vi "Julian Day_subVI.vi"() -> (0 "second":dbl, 1 "minute":dbl, 2 "hour":dbl, 3 "Julian Day":dbl format="%#_8g")   [LabVIEW 2019]
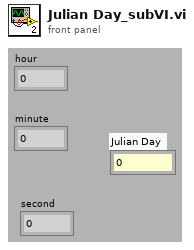
[diagram p1: front panel]
types:
  T1 = cluster{"second":i32, "minute":i32, "hour":i32, "day of month":i32, "month":i32, "year":i32, "day of week":i32, "day of year":i32, "is DST":i32}
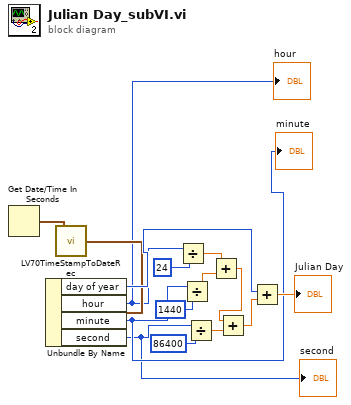
[diagram p0: block diagram]
diagram:
  n1 = Get Date/Time In Seconds() -> (seconds since 1Jan1904=w5:timestamp)
  n2 = call <vilib>:"LV70TimeStampToDateRec.vi"("time stamp"=w5) -> ("date time rec"=w6:T1)
  n3 = Unbundle By Name(w6) -> ("day of year"=w15:i32, "hour"=w3:i32, "minute"=w2:i32, "second"=w1:i32)
  "hour" <- w3
  "minute" <- w2
  "second" <- w1
  n4 = Divide(x=w3, y=24) -> (x/y=w12:dbl)
  n5 = Divide(x=w2, y=1440) -> (x/y=w10:dbl)
  n6 = Divide(x=w1, y=86400) -> (x/y=w11:dbl)
  n7 = Add(x=w12, y=w10) -> (x+y=w13:dbl)
  n8 = Add(x=w13, y=w11) -> (x+y=w14:dbl)
  n9 = Add(x=w15, y=w14) -> (x+y=→"Julian Day":dbl)
